vi "PKG_IMC_SetGantry.vi"(6 "axis":i32, 7 "maxis":i32, 9 "limit":u16, 10 "gantrykp":dbl, 11 "handle":u32) -> (2 "function return":i32, 3 "handle out":u32)   [LabVIEW 2011, in "IMC_Pkg4xxx.lvlib"]
doc: "PKG_IMC_SetGantry(IMC_HANDLE handle, double gantrykp, unsigned short limit, int maxis, int axis);"
uses:
  IMC_Pkg4xxx.lvlib
  IMC_Pkg4xxx.dll
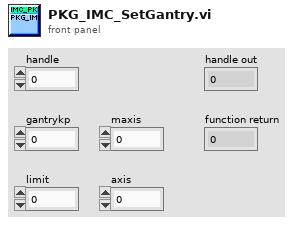
[diagram p1: front panel]
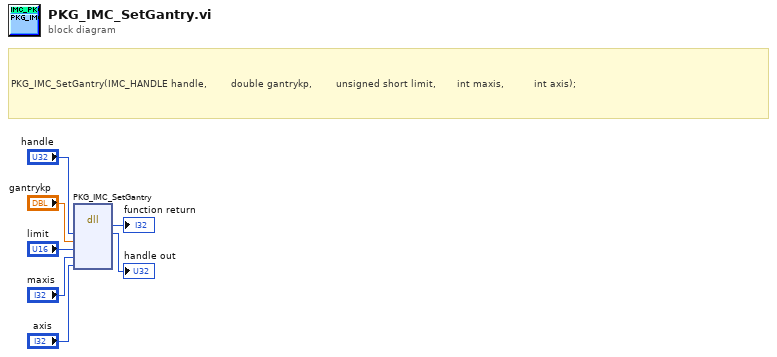
[diagram p0: block diagram]
diagram:
  # "PKG_IMC_SetGantry(IMC_HANDLE handle,  \t\t\t\t\t\tdouble gantrykp, \t\t\t\t\t\t\tunsigned short limit, \t\t\t\t\t\tint maxis, \t\t\t\t\t\t\t\t\tint axis);"
  n1 = dll-call lib="PTH1mabs F光盘刻录\niMC MotionIMCNet_V4.0IMCAppincLabviewIMC_PKG4xxxIMC_PKG4xxx\nIMC_Pkg4xxx.*" fn="PKG_IMC_SetGantry"("handle"="handle", "gantrykp"="gantrykp", "limit"="limit", "maxis"="maxis", "axis"="axis") -> (→"function return":i32, "handle"=→"handle out":u32)  [unwired: 7 in, 2 out]
